vi "File IO - Load Test Parameters from File.vi"(8 "error in (no error)":errorcluster, 10 "Parameter Definition File":path, 11 "Paramater Value File":path) -> (0 "error out":errorcluster, 2 "Experiment Parameter Values":T1(array[cluster]))   [LabVIEW 2012, in "Core SubVIs.lvlib"]
uses:
  Core SubVIs.lvlib
  <vilib>/Utility/config.llb/Read Key (String).vi
  <vilib>/Utility/config.llb/NI_LVConfig.lvlib
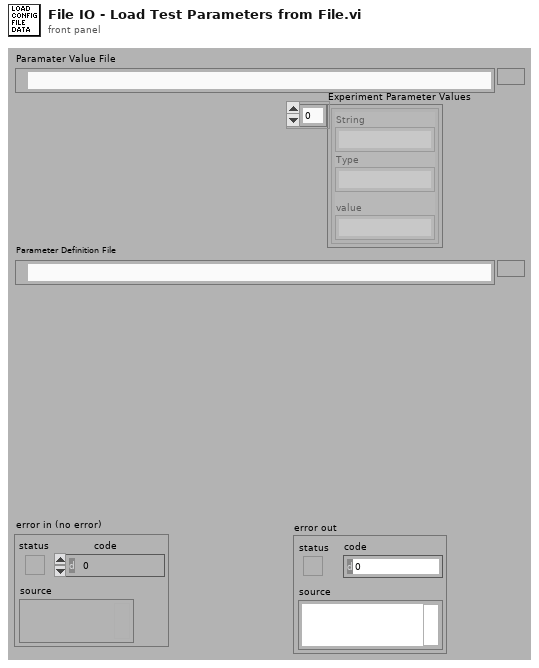
[diagram p1: front panel]
types:
  T1 = cluster{"String":string, "Type":string, "value":string}[]
  T2 = typedef "NI_LVConfig.lvlib/Config Data RefNum.ctl" = refnum<k1>
  T3 = cluster{"String":string, "value":string, "value":string}
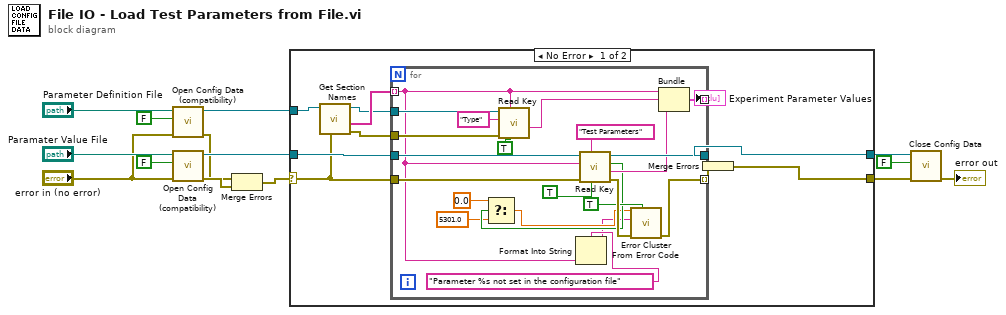
[diagram p0: block diagram]
diagram:
  n1 = call <vilib>:"Open Config Data (compatibility).vi"("error in (no error)"="error in (no error)", "create file if necessary (T)"=FALSE ("create file if necessary? (T)"), "configuration file path"="Parameter Definition File") -> ("error out"=w1:errorcluster, "refnum"=w2:T2)  [unwired: 6 in, 1 out]
  n2 = call <vilib>:"Open Config Data (compatibility).vi"("error in (no error)"="error in (no error)", "create file if necessary (T)"=FALSE ("create file if necessary? (T)"), "configuration file path"="Paramater Value File") -> ("error out"=w4:errorcluster, "refnum"=w12:T2)  [unwired: 6 in, 1 out]
  n3 = Merge Errors(w1, w4) -> (w3:errorcluster)
  n4 = case shown="No Error" w3 {
    selector: w3 -> [w18 w48]
    tunnel: w12 -> [w20 w47]
    tunnel: [w23 w48] -> w9
    tunnel: [w22 w47] -> w10
    tunnel: w2 -> [w19 _]
    frame No Error {
      n5 = call <vilib>:"Get Section Names.vi"("error in (no error)"=w18, "refnum"=w19) -> ("error out"=w15:errorcluster, "section names"=w17:string[], "refnum out"=w16:T2)  [unwired: 7 out]
      n6 = for {
        tunnel: w17 -> [w26] mode=indexing
        tunnel: w20 -> [w46]
        tunnel: w18 -> [w45]
        tunnel: [w32] -> w24 mode=indexing
        tunnel: [w44] -> w22
        tunnel: [w41] -> w21 mode=indexing
        tunnel: w16 -> [w39]
        tunnel: w15 -> [w40]
        n7 = call-poly <vilib>:"Read Key.vi"("read raw string? (F)"=TRUE, "section"=w26, "error in (no error)"=w40, "key"="Type", "refnum"=w39) -> ("value"=w36:string)  [unwired: 1 in, 5 out]
        n8 = Format Into String(format string="Parameter %s not set in the configuration file" ("error message (\"\")"), w26) -> (resulting string=w25:string)  [unwired: 2 in, 1 out]
        n9 = call-poly <vilib>:"Read Key.vi"("read raw string? (F)"=TRUE, "section"="Test Parameters", "error in (no error)"=w45, "key"=w26, "refnum"=w46) -> ("error out"=w34:errorcluster, "value"=w35:string, "found?"=w30:bool, "refnum out"=w44:T2)  [unwired: 1 in, 2 out]
        n10 = Select(t=0.0, s=w30, f=5301.0) -> (s? t:f=w28:dbl)
        n11 = call <vilib>:"Error Cluster From Error Code.vi"("show call chain? (False)"=TRUE, "error in (no error)"=w34, "error message (\"\")"=w25, "error code (0)"=w28) -> ("error out"=w32:errorcluster)  [unwired: 5 out]
        n12 = Bundle("String"=w26, "value"=w36, "value"=w35) -> (w41:T3)  [unwired: 1 out]
      }
      "Experiment Parameter Values" <- w21
      n13 = Merge Errors(w24) -> (w23:errorcluster)
    }
    frame Error {
    }
  }
  n14 = call <vilib>:"Close Config Data.vi"("error in (no error)"=w9, "write file if changed (T)"=FALSE ("write configuration file? (T)"), "refnum"=w10) -> ("error out"=→"error out":errorcluster)  [unwired: 8 out]
